vi "test_fpga_pid.vi"() -> ()   [LabVIEW 2016]
uses:
  <vilib>/Platform/TimedLoop/XDataNode/timing_clust.ctl
  <vilib>/Platform/TimedLoop/XDataNode/nitl_modes.ctl
  <vilib>/Platform/TimedLoop/XDataNode/wakeup.ctl
  <vilib>/rvi/Emulation/niFpgaSctlEmulationGetInTimedLoop.vi
  <vilib>/rvi/Emulation/niFpgaEmulationReportErrorSimple.vi
  <vilib>/rvi/Emulation/niFpgaGetClockAttributes.vi
  <vilib>/rvi/Emulation/niFpgaCriticalErrorInLSC.vi
  <vilib>/Platform/TimedLoop/XDataNode/XDataNode.xnode
  <vilib>/Platform/TimedLoop/XDataNode/XDNodeRunTimeDep.lvlib
panel:
  out "ready for input":bool
  out "output":T1
  out "output valid":bool
  in  "input":fxp<+/-,24,16>
  in  "fbParams":T2={"enable"=FALSE, "setPoint"=0.001007080078125, "pGain"=0.0, "iGain"=0.10000038146972656, "gainScale"=0}
  in  "liftOffParams":T3={"liftHeight"=0.0498046875, "disengagePos"=-1.0, "liftOff"=FALSE} {"disengagePos" format="%#_28g"}
  in  "input valid":bool=TRUE
  in  "manualMotion":T4
  in  "ready for output (T)":bool=TRUE
  in  "limits":T5={"upperLimit"=2.0, "lowerLimit"=0.0}
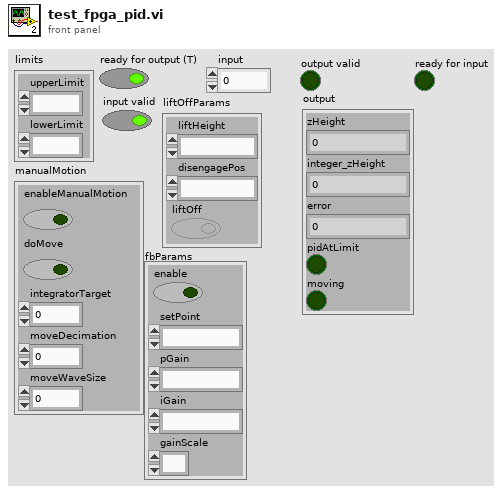
[diagram p1: front panel]
types:
  T1 = cluster{"zHeight":fxp<+/-,28,1>, "integer_zHeight":i16, "error":fxp<+/-,25,2>, "pidAtLimit":bool, "moving":bool}
  T2 = cluster{"enable":bool, "setPoint":fxp<+/-,17,1>, "pGain":fxp<+/-,20,4>, "iGain":fxp<+/-,20,1>, "gainScale":i8}
  T3 = cluster{"liftHeight":fxp<+/-,15,4>, "disengagePos":fxp<+/-,22,1>, "liftOff":bool}
  T4 = cluster{"enableManualMotion":bool, "doMove":bool, "integratorTarget":fxp<+/-,22,2>, "moveDecimation":u16, "moveWaveSize":u16}
  T5 = cluster{"upperLimit":fxp<+/-,28,4>, "lowerLimit":fxp<+/-,28,4>}
  T6 = typedef "XDNodeRunTimeDep.lvlib/timing_clust.ctl" = cluster{"Expected End [f-1]":u64, "Actual End [f-1]":u64, "Finished Late? [f-1]":bool, "Expected End [i-1]":u64, "Actual End [i-1]":u64, "Finished Late? [i-1]":bool, "Expected Start [i]":u64, "Actual Start [i]":u64, "Expected Start [f]":u64, "Actual Start [f]":u64, "Source Name":string, "Structure Name":string, "Period":i64, "Deadline":i64, "Offset":i64, "Start":i64, "Priority":i32, "Timeout":i32, "Mode":T7, "Wakeup Reason":T8, "Error":errorcluster, "Source Type":string, "Secondary Source Type":string, "Global End Time":u64, "Global Start Time":u64, "Frame Duration":u64, "Iteration Duration":u64, "Assigned CPU":i32, "I/O Scan Engine Mode":u32}
  T7 = typedef "XDNodeRunTimeDep.lvlib/nitl_modes.ctl" = enum32{"No Change", "Process missed periods, maintain original phase", "Discard missed periods, maintain original phase", "Process missed periods, ignore original phase", "Discard missed periods, ignore original phase"}
  T8 = typedef "XDNodeRunTimeDep.lvlib/wakeup.ctl" = enum32{"Normal", "Aborted", "Asynchronous wakeup", "Timing source error", "Timed loop error", "Timeout"}
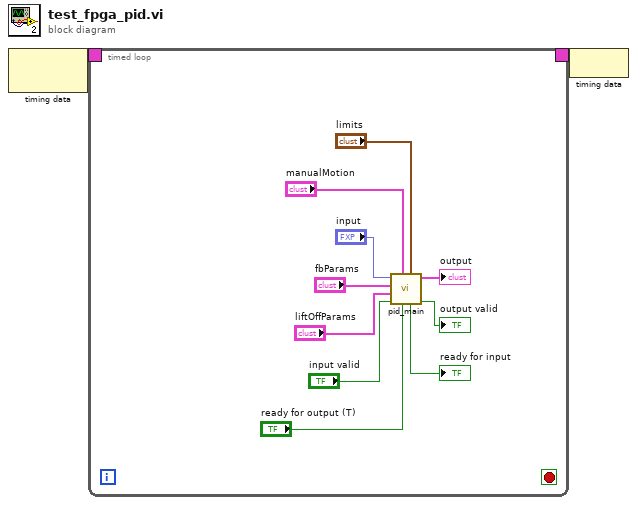
[diagram p0: block diagram]
diagram:
  n1 = node-c288() -> (w2:T6)  [unwired: 1 in]
  n2 = timed-loop {
    timing: w2 -> [_]
    timing-out: [_] -> w1
    stop <- _ stop-if-true
    n3 = call "pid_main.vi"("limits"="limits", "ready for output (T)"="ready for output (T)", "manualMotion"="manualMotion", "input valid"="input valid", "liftOffParams"="liftOffParams", "fbParams"="fbParams", "input"="input") -> ("output valid"=→"output valid":bool, "output"=→"output":T1, "ready for input"=→"ready for input":bool)  [unwired: 2 in]
  }
  n4 = node-c288(w1) -> ()
